vi "calculator.vi"() -> ()   [LabVIEW 2021]
panel:
  out "Display":string
  out "Number of Matches Second Form":i32=7
  out "Number of Matches First Form":i32=7
  in  "Calculator UI":T1
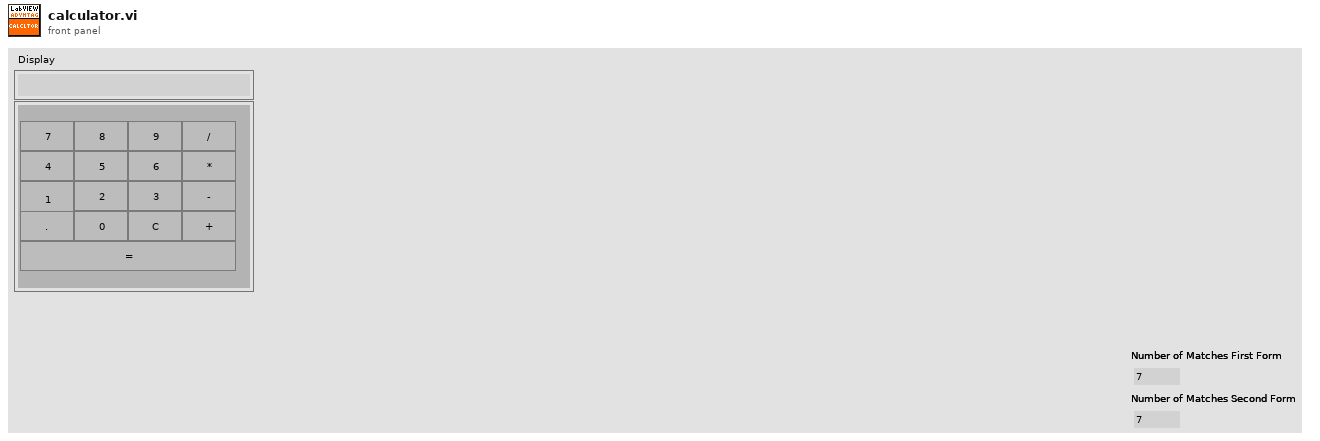
[diagram p1: front panel]
types:
  T1 = cluster{"1":bool, "2":bool, "3":bool, "Add":bool, "4":bool, "5":bool, "6":bool, "Subtract":bool, "7":bool, "8":bool, "9":bool, "Result":bool, "0":bool, "Multiply":bool, "Divide":bool, ".":bool, "C":bool}
  T2 = enum16{"No Function", "Add", "Subtract", "Multiply", "Divide"}
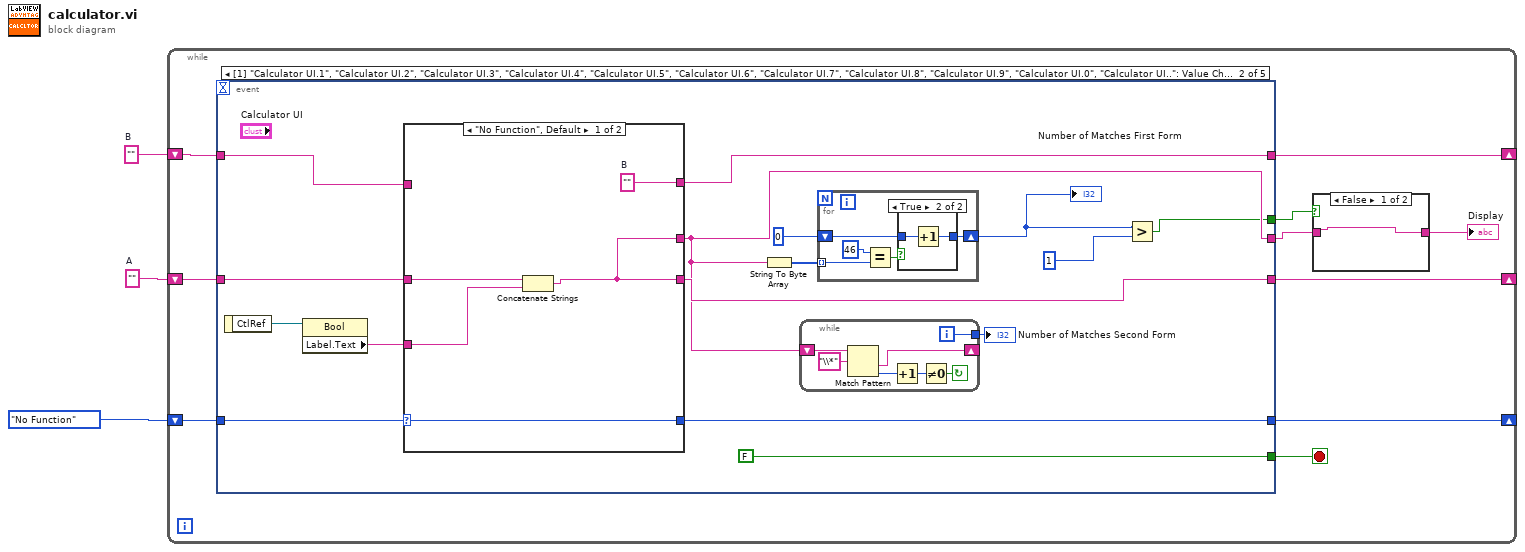
[diagram p0: block diagram]
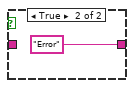
[diagram p2: hidden frame]
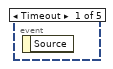
[diagram p3: hidden frame]
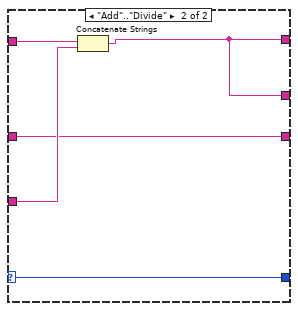
[diagram p5: hidden frame]
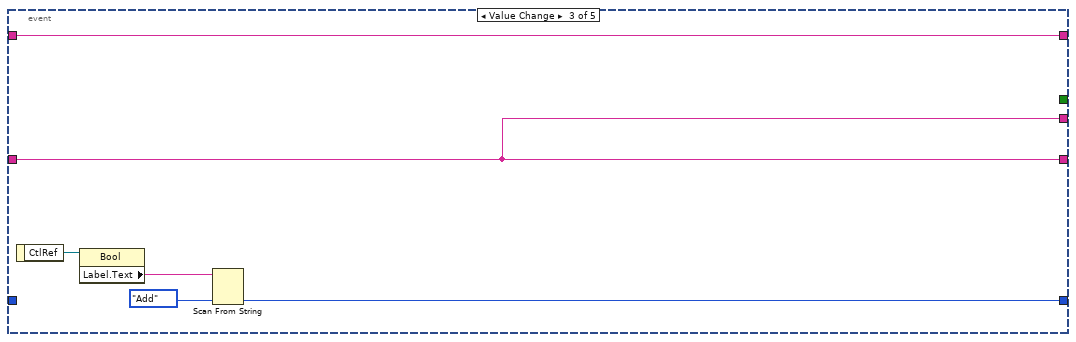
[diagram p6: hidden frame]
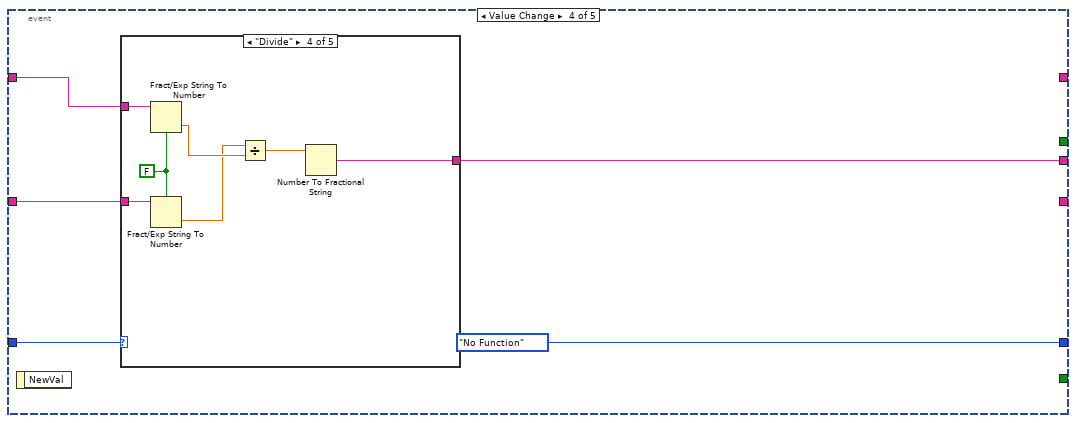
[diagram p7: hidden frame]
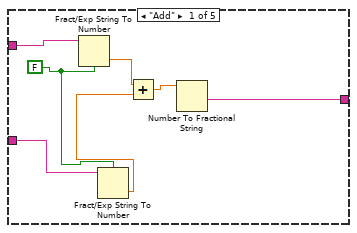
[diagram p8: hidden frame]
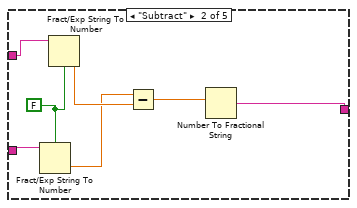
[diagram p9: hidden frame]
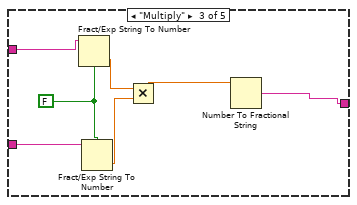
[diagram p10: hidden frame]
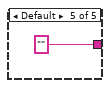
[diagram p11: hidden frame]
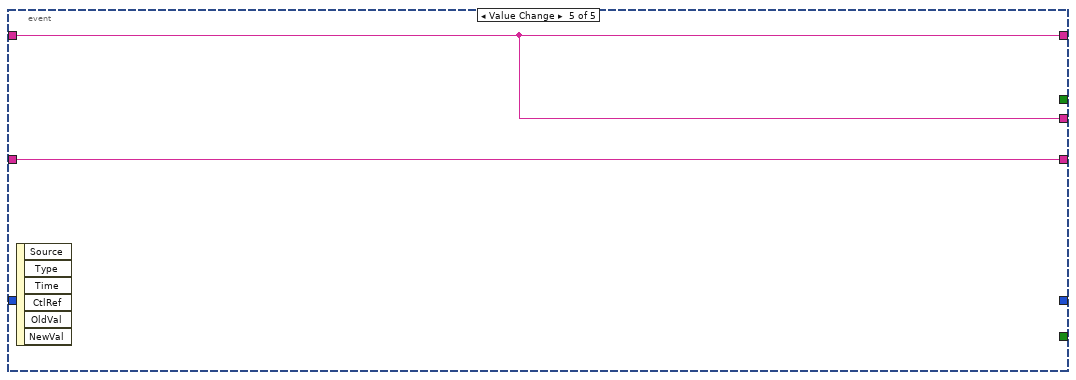
[diagram p12: hidden frame]
diagram:
  w2 = ""  # A
  w3 = ""  # B
  n1 = while {
    shift-right: [w9] -> _
    shift-left: w3 -> [w12]
    shift-right: [w8] -> _
    shift-left: w2 -> [w13]
    shift-right: [w10] -> _
    shift-left: T2."No Function" -> [w11]
    stop <- w7 stop-if-true
    n2 = event shown="[1] \"Calculator UI.1\", \"Calculator UI.2\", \"Calculator UI.3\", \"Calculator UI.4\", \"Calculator UI.5\", \"Calculator UI.6\", \"Calculator UI.7\", \"Calculator UI.8\", \"Calculator UI.9\", \"Calculator UI.0\", \"Calculator UI..\": Value Change" {
      selector: _ -> [_ _ _ _ _]
      dyn-events: _ -> [_ _ _ _ _]
      timeout: _ -> [_ _ _ _ _]
      tunnel: w13 -> [_ w29 w57 w64 w97]
      tunnel: w12 -> [_ w23 w62 w65 w98]
      tunnel: w11 -> [_ w30 _ w67 _]
      tunnel: [_ w27 w58 T2."No Function" _] -> w10
      tunnel: [_ w26 w62 _ w98] -> w9
      tunnel: [_ w25 w57 _ w97] -> w8
      tunnel: [_ FALSE _ _ _] -> w7
      tunnel: [_ w19 w57 w63 w98] -> w5
      tunnel: [_ w16 _ _ _] -> w6
      event Timeout {
        n3 = event-data() -> ()  [unwired: 1 in, 1 out]
      }
      event "Calculator UI.1", "Calculator UI.2", "Calculator UI.3", "Calculator UI.4", "Calculator UI.5", "Calculator UI.6", "Calculator UI.7", "Calculator UI.8", "Calculator UI.9", "Calculator UI.0", "Calculator UI..": Value Change {
        n4 = event-data() -> ("CtlRef"=w31:refnum<vi>)  [unwired: 1 in]
        n5 = property class="Bool"(reference=w31) -> ("Label.Text"=w28:string)  [unwired: 1 in, 2 out]
        n6 = case shown="\"No Function\", Default" w30 {
          selector: w30 -> [w49 w53]
          tunnel: w29 -> [w51 w54]
          tunnel: w28 -> [w50 w55]
          tunnel: [w49 w53] -> w27
          tunnel: [w48 w52] -> w26
          tunnel: [w47 w54] -> w25
          tunnel: w23 -> [_ w56]
          tunnel: [w47 w52] -> w19
          frame "No Function", Default {
            w48 = ""  # B
            n7 = Concatenate Strings(w51, w50) -> (w47:string)
          }
          frame "Add".."Divide" {
            n8 = Concatenate Strings(w56, w55) -> (w52:string)
          }
        }
        n9 = String To Byte Array(string=w19) -> (unsigned byte array=w21:u8[])
        n10 = while {
          tunnel: [w32] -> w20
          shift-left: w19 -> [w38]
          shift-right: [w36] -> _
          i -> [w32]
          stop <- w33 continue-if-true
          n11 = Match Pattern(string=w38, regular expression="\\*") -> (after substring=w36:string, offset past match=w35:i32)  [unwired: 1 in, 2 out]
          n12 = Increment(x=w35) -> (x+1=w34:i32)
          n13 = Not Equal To 0?(x=w34) -> (x != 0?=w33:bool)
        }
        "Number of Matches Second Form" <- w20
        n14 = for {
          shift-right: [w41] -> w18
          shift-left: 0 -> [w42]
          tunnel: w21 -> [w40] mode=indexing
          n15 = Equal?(x=u8 46, y=w40) -> (x = y?=w43:bool)
          n16 = case shown="True" w43 {
            tunnel: w42 -> [w44 w46]
            tunnel: [w44 w45] -> w41
            frame False {
            }
            frame True {
              n17 = Increment(x=w46) -> (x+1=w45:i32)
            }
          }
        }
        "Number of Matches First Form" <- w18
        n18 = Greater?(x=w18, y=1) -> (0:w16:bool)
      }
      event "Calculator UI.Add", "Calculator UI.Subtract", "Calculator UI.Multiply", "Calculator UI.Divide": Value Change {
        n19 = event-data() -> ("CtlRef"=w61:refnum<vi>)  [unwired: 1 in]
        n20 = property class="Bool"(reference=w61) -> ("Label.Text"=w59:string)  [unwired: 1 in, 2 out]
        n21 = Scan From String "Scan From String"(input string=w59, default 1=T2."Add") -> (output 1=w58:T2)  [unwired: 3 in, 3 out]
      }
      event "Calculator UI.Result": Value Change {
        n22 = event-data() -> ()  [unwired: 1 in, 1 out]
        n23 = case shown="\"Divide\"" w67 {
          tunnel: w65 -> [w71 w81 w88 w95 _]
          tunnel: w64 -> [w73 w80 w87 w94 _]
          tunnel: [w74 w78 w84 w90 ""] -> w63
          frame "Add" {
            w68 = FALSE
            n24 = Fract/Exp String To Number(use system decimal point (T)=w68, string=w71) -> (number=w70:dbl)  [unwired: 2 in, 1 out]
            n25 = Fract/Exp String To Number(use system decimal point (T)=w68, string=w73) -> (number=w72:dbl)  [unwired: 2 in, 1 out]
            n26 = Add(x=w70, y=w72) -> (x+y=w69:dbl)
            n27 = Number To Fractional String(number=w69) -> (F-format string=w74:string)  [unwired: 3 in]
          }
          frame "Subtract" {
            w77 = FALSE
            n28 = Fract/Exp String To Number(use system decimal point (T)=w77, string=w80) -> (number=w75:dbl)  [unwired: 2 in, 1 out]
            n29 = Fract/Exp String To Number(use system decimal point (T)=w77, string=w81) -> (number=w76:dbl)  [unwired: 2 in, 1 out]
            n30 = Subtract(x=w75, y=w76) -> (x-y=w79:dbl)
            n31 = Number To Fractional String(number=w79) -> (F-format string=w78:string)  [unwired: 3 in]
          }
          frame "Multiply" {
            w82 = FALSE
            n32 = Fract/Exp String To Number(use system decimal point (T)=w82, string=w88) -> (number=w86:dbl)  [unwired: 2 in, 1 out]
            n33 = Fract/Exp String To Number(use system decimal point (T)=w82, string=w87) -> (number=w85:dbl)  [unwired: 2 in, 1 out]
            n34 = Multiply(x=w86, y=w85) -> (x*y=w83:dbl)
            n35 = Number To Fractional String(number=w83) -> (F-format string=w84:string)  [unwired: 3 in]
          }
          frame "Divide" {
            w89 = FALSE
            n36 = Fract/Exp String To Number(use system decimal point (T)=w89, string=w95) -> (number=w93:dbl)  [unwired: 2 in, 1 out]
            n37 = Fract/Exp String To Number(use system decimal point (T)=w89, string=w94) -> (number=w92:dbl)  [unwired: 2 in, 1 out]
            n38 = Divide(x=w92, y=w93) -> (x/y=w91:dbl)
            n39 = Number To Fractional String(number=w91) -> (F-format string=w90:string)  [unwired: 3 in]
          }
          frame Default {
          }
        }
      }
      event "Calculator UI.C": Value Change {
        n40 = event-data() -> ()  [unwired: 1 in, 6 out]
      }
    }
    n41 = case shown="False" w6 {
      tunnel: w5 -> [w14 _]
      tunnel: [w14 "Error" ("Display 2")] -> w4
      frame False {
      }
      frame True {
      }
    }
    "Display" <- w4
  }
